vi "ServiceWatchDog.vi"(8 "error in (no error)":errorcluster, 11 "NHRGridSim in":refnum<class "NHRGridSim.lvclass">) -> (0 "error out":errorcluster, 3 "NHRGridSim out":refnum<class "NHRGridSim.lvclass">)   [LabVIEW 2018, in "AcPwrPlugins.lvlib" / "NHRGridSim.lvclass"]
uses:
  NHRGridSim.lvclass
  <instrlib>/NH Research 9400 Series/NH Research 9400 Series.lvlib
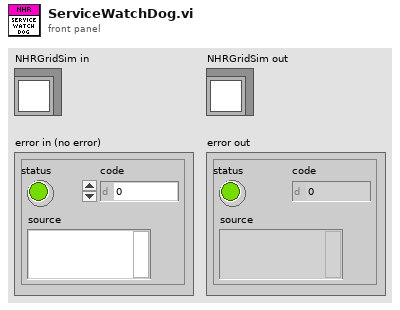
[diagram p1: front panel]
types:
  T1 = typedef "AcPwrPlugins.lvlib/NHRGridSim.lvclass/Modules.ctl" = cluster{"Measurement":cluster{"ApertureLength (s)":dbl, "NumberOfSamples":u32}, "Ranges":cluster{"Irange (A)":dbl, "Vrange (V)":dbl}, "Mode":u8, "TransformerRatio":dbl, "Handle":string, "FreqOut (Hz)":dbl, "Connected":bool, "btnIdQuery":bool, "btnReset":bool, "Initialize Timeout ( ms)":u32, "Phase (0: All)":i32, "Grid (0: Normal)":i32, "WatchDog":cluster{"Enable WatchDog":bool, "Robust WatchDog":bool, "Watchdog Interval (s)":dbl}, "Safety Limits":cluster{"Min Voltage (V)":dbl, "Min Voltage Time (s)":dbl, "Max Voltage (V)":dbl, "MaxVoltage Time (s)":dbl, "Max Source Amps (A)":dbl, "Max Source Amps Time (s)":dbl, "Max Sink Amps (A)":dbl, "Max Sink Amps Time (s)":dbl, "Max Source Power (W)":dbl, "Max Source Power Time (s)":dbl, "Max Sink Power (W)":dbl, "Max Sink Power Time (s)":dbl, "Peak Voltage (V)":dbl, "Peak Voltage Enable":bool, "Peak Amps (A)":dbl, "Peak Amps Enable":bool}, "Phases":cluster{"Pout (W)":dbl, "Iout (A)":dbl, "PhaseAngle":dbl, "Vout (V)":dbl, "Phase Name":string}[]}[]
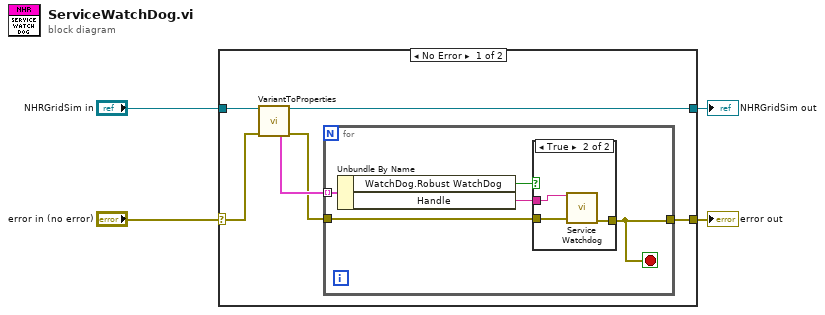
[diagram p0: block diagram]
diagram:
  n1 = case shown="No Error" "error in (no error)" {
    selector: "error in (no error)" -> [w9 w21]
    tunnel: [w5 w21] -> w3
    tunnel: [w8 w20] -> w2
    tunnel: "NHRGridSim in" -> [w10 w20]
    frame No Error {
      n2 = call "VariantToProperties.vi"("NHRGridSim in"=w10, "error in (no error)"=w9) -> ("NHRGridSim out"=w8:refnum<class "NHRGridSim.lvclass">, "Modules"=w7:T1, "error out"=w6:errorcluster)  [unwired: 7 in, 4 out]
      n3 = for {
        tunnel: w7 -> [w15] mode=indexing
        tunnel: w6 -> [w12]
        tunnel: [w11] -> w5
        stop <- w11 stop-if-true
        n4 = Unbundle By Name(w15) -> ("WatchDog.Robust WatchDog"=w14:bool, "Handle"=w13:string)
        n5 = case shown="True" w14 {
          tunnel: w13 -> [_ w18]
          tunnel: w12 -> [w16 w19]
          tunnel: [w16 w17] -> w11
          frame False {
          }
          frame True {
            n6 = call <instrlib>:"Service Watchdog.vi"("VISA resource name"=w18, "error in (no error)"=w19) -> ("error out"=w17:errorcluster)  [unwired: 12 in, 1 out]
          }
        }
      }
    }
    frame Error {
    }
  }
  "error out" <- w3
  "NHRGridSim out" <- w2
